vi "Error Message.vi"(8 "error in (no error)":errorcluster {"code" format="%.0x"}, 10 "Error Code":i32 format="%.0g", 11 "instrument handle":refnum<k15>) -> (0 "error out":errorcluster {"code" format="%.0x"}, 2 "Error Message":string, 3 "instrument handle out":refnum<k15>)   [LabVIEW 2014, in "Agilent NA.lvlib"]
doc: "Translates the error return value from an IVI driver VI to a user-readable string. The user should pass a buffer with at least 256 bytes for the ErrorMessage parameter."
uses:
  Agilent NA.lvlib
  AgNA.dll
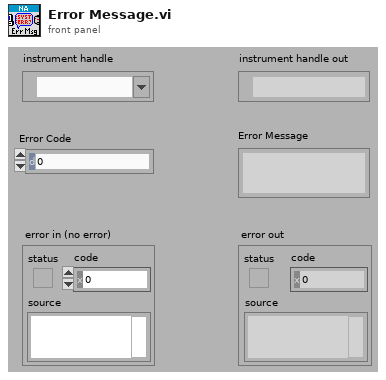
[diagram p1: front panel]
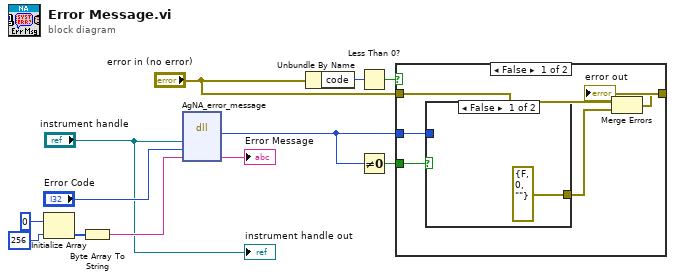
[diagram p0: block diagram]
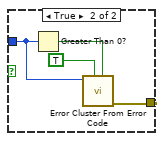
[diagram p2: hidden frame]
diagram:
  n1 = Initialize Array(u8 0, 256) -> (w7:u8[])
  n2 = Byte Array To String(unsigned byte array=w7) -> (string=w11:string)
  n3 = dll-call lib="AgNA**.dll" fn="AgNA_error_message" label="error_message"("instrument handle", "Error Code", w11) -> (w2:i32, →"Error Message":string)  [unwired: 4 in, 3 out]
  n4 = Unbundle By Name("error in (no error)") -> ("code"=w6:i32)
  n5 = Less Than 0?(x=w6) -> (x < 0?=w4:bool)
  n6 = Not Equal To 0?(x=w2) -> (x != 0?=w3:bool)
  n7 = case shown="False" w4 {
    tunnel: [w14 w24] -> w1
    tunnel: w3 -> [w18 _]
    tunnel: "error in (no error)" -> [w16 w24]
    tunnel: w2 -> [w17 _]
    frame False {
      n8 = case shown="False" w18 {
        tunnel: w17 -> [_ w21]
        tunnel: [errorcluster {"status"=FALSE, "code"=0, "source"=""} ("error out") w20] -> w15
        frame False {
        }
        frame True {
          n9 = Greater Than 0?(x=w21) -> (x > 0?=w22:bool)
          n10 = call "Error Cluster From Error Code.vi"("is warning? (False)"=w22, "show call chain? (False)"=TRUE, "error code (0)"=w21) -> ("error out"=w20:errorcluster)  [unwired: 1 in, 5 out]
        }
      }
      n11 = Merge Errors(w16, w15) -> (w14:errorcluster)
    }
    frame True {
    }
  }
  "error out" <- w1
  "instrument handle out" <- "instrument handle"
